vi "Image Acquistion Dynamic.vi"(7 "lpszRefPath":string, 8 "error in (no error)":errorcluster, 9 "nMode":u32, 10 "pRefImage":u16, 11 "nSensorIP":u32) -> (0 "error out":errorcluster, 2 "pRefImage out":u16, 3 "function return":i32, 5 "lpszRefPath out":string)   [LabVIEW 2017, in "imgAcquisition.lvlib"]
doc: "DLLFunction int __stdcall ImageCapImageAcquistion_Dynamic(unsigned int nSensorIP, unsigned short** pRefImage, unsigned int nMode, LPCTSTR lpszRefPath);"
uses:
  imgAcquisition.lvlib
  lib/ImageCaptureDLL.dll
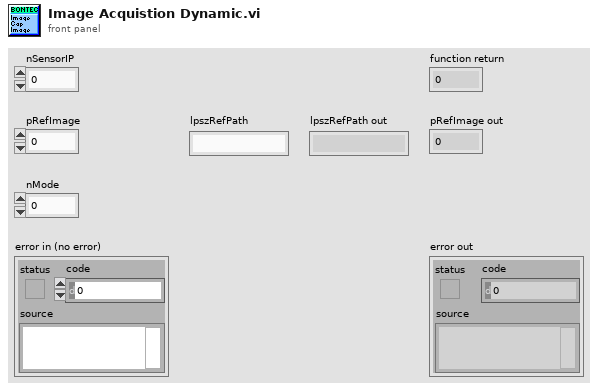
[diagram p1: front panel]
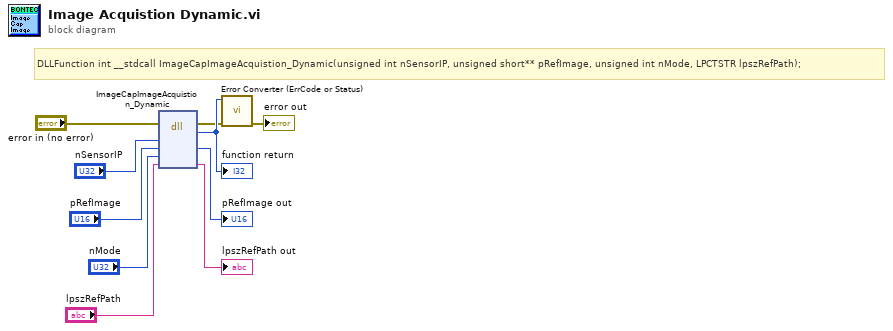
[diagram p0: block diagram]
diagram:
  # "DLLFunction int __stdcall ImageCapImageAcquistion_Dynamic(unsigned int nSensorIP, unsigned short** pRefImage, unsigned int nMode, LPCTSTR lpszRefPath);"
  n1 = dll-call lib="F:/BonTechFlatPanelLVDriver/lib/ImageCaptureDLL.*" fn="ImageCapImageAcquistion_Dynamic"(error in="error in (no error)", "nSensorIP"="nSensorIP", "pRefImage"="pRefImage", "nMode"="nMode", "lpszRefPath"="lpszRefPath") -> (error out=w2:errorcluster, w10:i32, "pRefImage"=→"pRefImage out":u16, "lpszRefPath"=→"lpszRefPath out":string)  [unwired: 4 in, 1 out]
  "function return" <- w10
  n2 = call "Error Converter (ErrCode or Status).vi"("error in (no error)"=w2, "error code"=w10) -> ("error out"=→"error out":errorcluster)  [unwired: 9 in]
